vi "실습 4-3 배열인덱스.vi"() -> ()   [LabVIEW 2014]
panel:
  out "원소 4":dbl=23312.0
  out "부분배열 2":dbl[](array[numeric])=[9.0, 8.0, 7.0, 6.0, 0.0, 0.0, 23312.0]
  out "부분배열":dbl[](array[numeric])=[3.0, 0.0, 7.0]
  in  "배열 2":dbl[][](array[numeric])=[[1.0, 0.0, 9.0], [2.0, 0.0, 8.0], [3.0, 0.0, 7.0], [4.0, 0.0, 6.0], [5.0, 0.0, 0.0], [6.0, 0.0, 0.0], [7.0, 0.0, 23312.0]]
  out "원소 3":dbl=3.0
  out "원소 2":dbl=2.0
  out "원소":dbl=1.0
  in  "배열":dbl[](array[numeric])=[1.0, 2.0, 3.0, 4.0, 5.0]
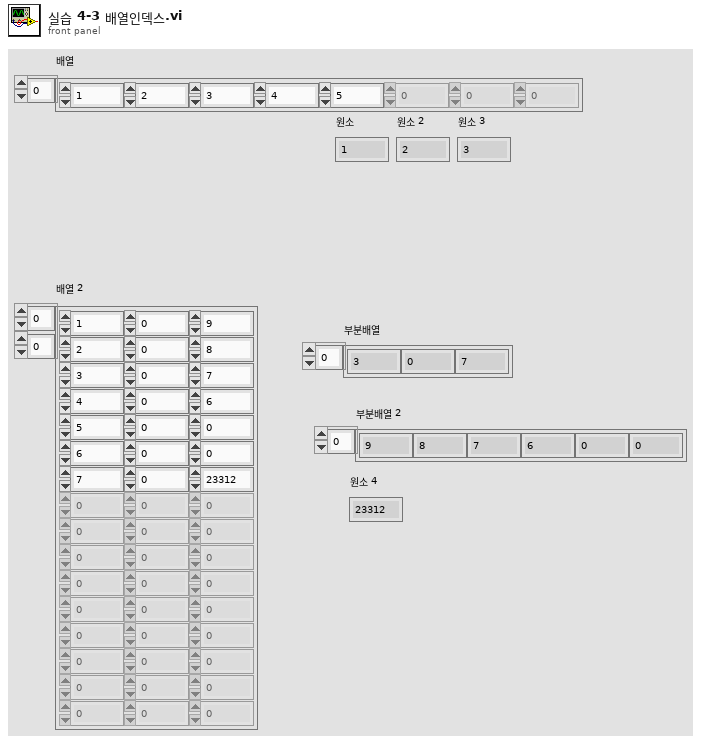
[diagram p1: front panel]
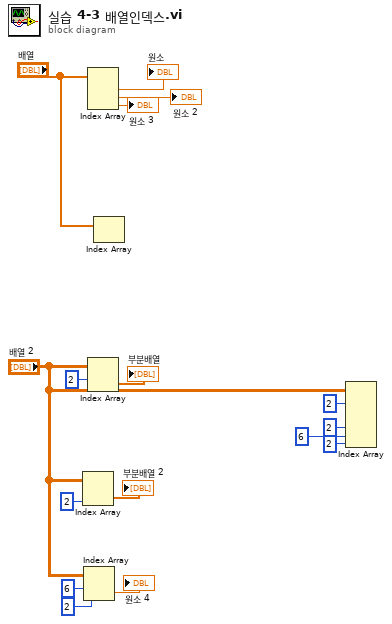
[diagram p0: block diagram]
diagram:
  n1 = Index Array(array="배열 2", index (col)=2 ("비활성화된 인덱스 (열)")) -> (element=→"부분배열 2":dbl[])  [unwired: 1 in]
  n2 = Index Array(array="배열 2", index (row)=6 ("인덱스 (행)"), index (col)=2 ("비활성화된 인덱스 (열)")) -> (element=→"원소 4":dbl)
  n3 = Index Array(array="배열") -> (element #1=→"원소":dbl, element #2=→"원소 2":dbl, element #3=→"원소 3":dbl)  [unwired: 3 in]
  n4 = Index Array(array="배열 2", index (row)=2 ("인덱스 (행)")) -> (element=→"부분배열":dbl[])  [unwired: 1 in]
  n5 = Index Array(array="배열") -> ()  [unwired: 1 in, 1 out]
  n6 = Index Array(array="배열 2", index (row) #1=2 ("인덱스 (행)"), index (col) #2=2 ("비활성화된 인덱스 (열)"), index (row) #3=6 ("비활성화된 인덱스 (행)"), index (col) #3=2 ("비활성화된 인덱스 (열)")) -> ()  [unwired: 2 in, 3 out]
